vi "PH_ImageStatistician.add new result.vi"(0 "i ref in":refnum<vi>, 2 "New Img Op Dataset":T1, 5 "error in (no error)":errorcluster) -> (14 "i ref out":refnum<vi>, 19 "error out":errorcluster)   [LabVIEW 2014, in "PH_ImageStatistician.lvlib"]
doc: "This VI investigates the new incoming data and adds them to the results already collected."
uses:
  PH_ImageStatistician.lvlib
  PH_ImageStatistician.Statistician Data.ctl
  PH_Common/PH_Common.lvlib
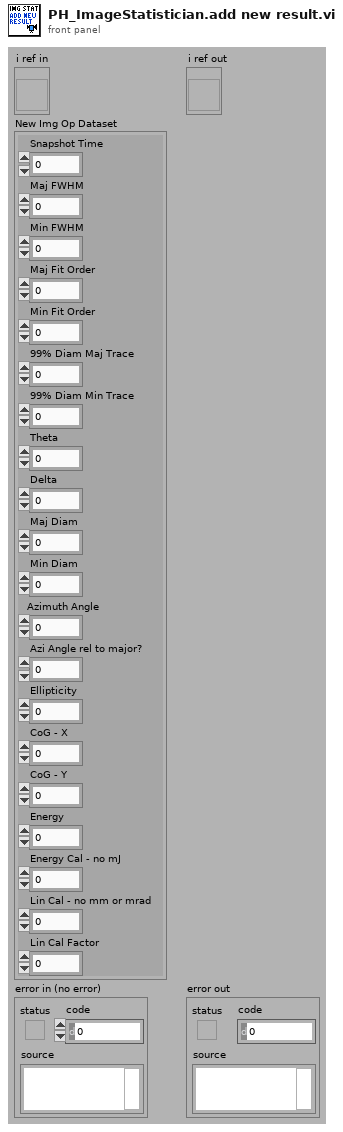
[diagram p1: front panel]
types:
  T1 = typedef "PH_ImageStatistician.lvlib/PH_ImageStatistician.Statistician Data.ctl" = cluster{"Snapshot Time":dbl, "Maj FWHM":dbl, "Min FWHM":dbl, "Maj Fit Order":dbl, "Min Fit Order":dbl, "99% Diam Maj Trace":dbl, "99% Diam Min Trace":dbl, "Theta":dbl, "Delta":dbl, "Maj Diam":dbl, "Min Diam":dbl, "Azimuth Angle":dbl, "Azi Angle rel to major?":dbl, "Ellipticity":dbl, "CoG - X":dbl, "CoG - Y":dbl, "Energy":dbl, "Energy Cal - no mJ":dbl, "Lin Cal - no mm or mrad":dbl, "Lin Cal Factor":dbl}
  T2 = typedef "PH_ImageStatistician.lvlib/PH_ImageStatistician.i attribute.ctl" = cluster{"GUI Refs ":cluster{"Status":refnum<vi>, "Result Graph":refnum<vi>, "Mean Data 1":refnum<vi>, "Std Dev Data 1":refnum<vi>, "Mean Data 2":refnum<vi>, "Std Dev Data 2":refnum<vi>, "Mean Data 3":refnum<vi>, "Std Dev Data 3":refnum<vi>, "Dummy Mean":refnum<vi>, "Dummy Std Dev":refnum<vi>, "Export Data":refnum<vi>, "Data 1":refnum<vi>, "Data 2":refnum<vi>, "Data 3":refnum<vi>, "Stat or Trend":refnum<vi>, "Delete":refnum<vi>, "Operator":refnum<vi>, "Start":refnum<vi>}, "Operator":string, "Data":T1[], "Stat or Trend":bool, "Data 1":T3, "Data 2":T3, "Data 3":T3, "Start":bool, "Datasets strored":i32, "Dataarray Size":i32}
  T3 = typedef "PH_ImageStatistician.lvlib/PH_ImageStatistician.select Data.ctl" = u16
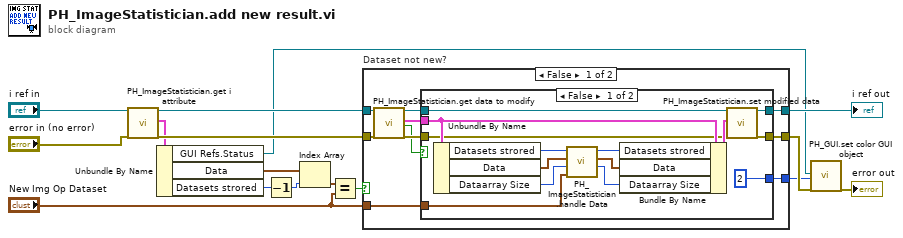
[diagram p0: block diagram]
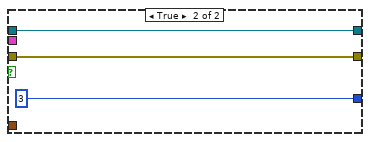
[diagram p2: hidden frame]
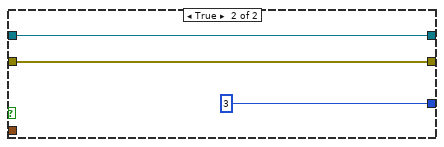
[diagram p3: hidden frame]
diagram:
  n1 = call "PH_ImageStatistician.get i attribute.vi"("i ref in"="i ref in", "error in (no error)"="error in (no error)") -> ("i ref out"=w12:refnum<vi>, "i attribute"=w11:T2, "error out"=w14:errorcluster)  [unwired: 15 in]
  n2 = Unbundle By Name(w11) -> ("GUI Refs.Status"=w8:refnum<vi>, "Data"=w4:T1[], "Datasets strored"=w1:i32)
  n3 = Decrement(x=w1) -> (x-1=w5:i32)
  n4 = Index Array(array=w4, index=w5) -> (element=w6:T1)
  n5 = Equal?(x=w6, y="New Img Op Dataset") -> (x = y?=w2:bool)
  n6 = case "Dataset not new?" shown="False" w2 {
    tunnel: [w23 w46] -> w15
    tunnel: w14 -> [w21 w45]
    tunnel: w12 -> [w20 w46]
    tunnel: [w19 w45] -> w9
    tunnel: [w18 3 ("status")] -> w7
    tunnel: "New Img Op Dataset" -> [w17 _]
    frame False {
      n7 = call "PH_ImageStatistician.get data to modify.vi"("i ref in"=w20, "error in (no error)"=w21) -> ("i ref out"=w24:refnum<vi>, "i attribute"=w26:T2, "timed out"=w22:bool, "error out"=w25:errorcluster)  [unwired: 14 in]
      n8 = case shown="False" w22 {
        tunnel: w26 -> [w33 _]
        tunnel: w25 -> [w32 w42]
        tunnel: [w39 w42] -> w19
        tunnel: w24 -> [w38 w43]
        tunnel: [w37 w43] -> w23
        tunnel: w17 -> [w28 _]
        tunnel: [2 ("status") 3] -> w18
        frame False {
          n9 = Unbundle By Name(w33) -> ("Datasets strored"=w27:i32, "Data"=w40:T1[], "Dataarray Size"=w36:i32)
          n10 = call "PH_ImageStatistician.handle Data.vi"("New Img Op Dataset"=w28, "Dataarray Size in"=w36, "Data in"=w40, "Datasets strored in"=w27) -> ("Dataarray Size out"=w34:i32, "Data out"=w29:T1[], "Datasets strored out"=w30:i32)  [unwired: 3 in]
          n11 = Bundle By Name(cluster=w33, "Datasets strored"=w30, "Data"=w29, "Dataarray Size"=w34) -> (w35:T2)
          n12 = call "PH_ImageStatistician.set modified data.vi"("i ref in"=w38, "i attribute"=w35, "error in (no error)"=w32) -> ("i ref out"=w37:refnum<vi>, "error out"=w39:errorcluster)  [unwired: 15 in]
        }
        frame True {
        }
      }
    }
    frame True {
    }
  }
  "i ref out" <- w15
  n13 = call "PH_GUI.set color GUI object.vi"("GUI object Ref"=w8, "State"=w7, "error in (no error)"=w9) -> ("error out"=→"error out":errorcluster)  [unwired: 16 in]
